vi "S8300E_BootupTime_Delay.vi"() -> ()   [LabVIEW 2011]
uses:
  Instance           3 28Saved   KT55_WaitBootUP_Time .vi
panel:
  out "Begin Time":u32
  out "倒數進度%":u8(slide) scale=0.0..100.0
  out "count down Sec":dbl
  out "系統定義到數秒數":string
  out "System Start Time":u32
  # "S8300E Wait for UUT Ready"
  # "2014-12-15"
  # "Wait for the system Ready\n系統需穩定後才能測試"
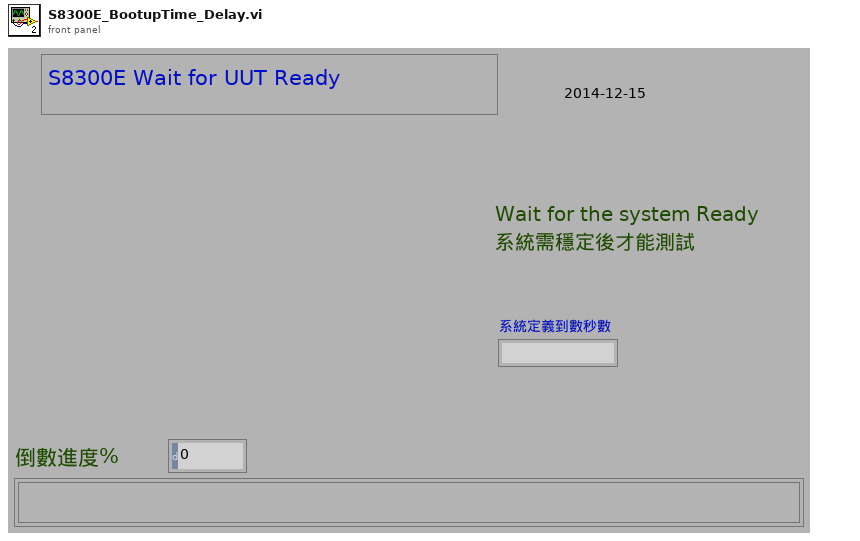
[diagram p1: front panel]
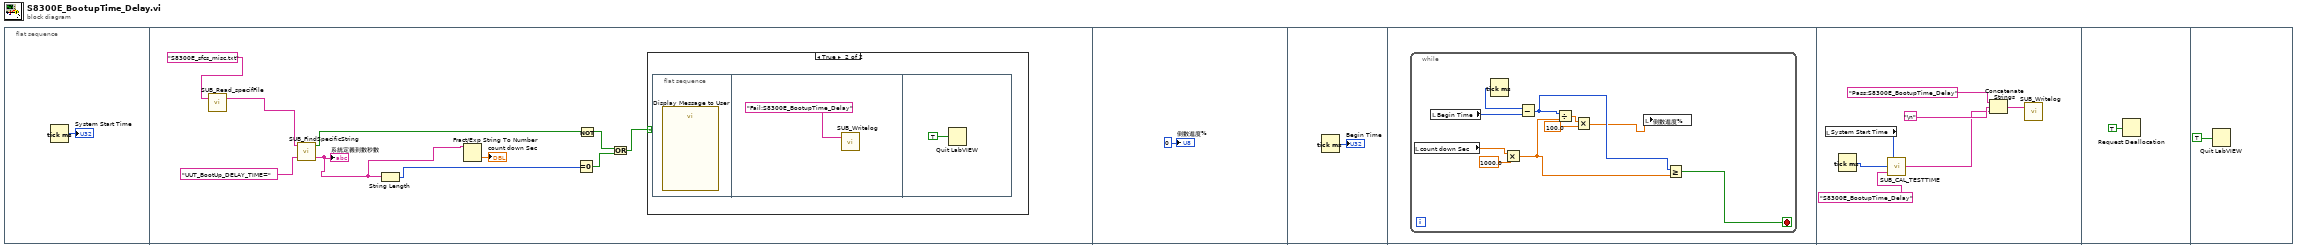
[diagram p0: block diagram]
diagram:
  n1 = flat-sequence {
    frame #0 {
      n2 = Tick Count (ms)() -> (millisecond timer value=→"System Start Time":u32)
    }
    frame #1 {
      n3 = call "SUB_Read_specifFile.vi"("name or relative path"="S8300E_sfcs_misc.txt" ("Script FileName")) -> ("text"=w2:string)  [unwired: 1 in, 1 out]
      n4 = call "SUB_FindSpecificString.vi"("Find this String"="UUT_BootUp_DELAY_TIME=" ("string"), "String data"=w2) -> ("before \"; \" string"=w10:string, "Found"=w7:bool)  [unwired: 2 in]
      "系統定義到數秒數" <- w10
      n5 = String Length(string=w10) -> (length=w8:i32)
      n6 = Fract/Exp String To Number(string=w10) -> (number=→"count down Sec":dbl)  [unwired: 3 in, 1 out]
      n7 = Equal To 0?(x=w8) -> (x = 0?=w5:bool)
      n8 = Not(x=w7) -> (.not. x?=w6:bool)
      n9 = Or(x=w6, y=w5) -> (x .or. y?=w4:bool)
      n10 = case shown="True" w4 {
        frame False {
        }
        frame True {
          n11 = flat-sequence {
            frame #0 {
              n12 = call "Display Message to User"() -> ()  [unwired: 10 in, 2 out]
            }
            frame #1 {
              n13 = call "SUB_Writelog.vi"("Pass/Fail"="Fail:S8300E_BootupTime_Delay") -> ()  [unwired: 2 in]
            }
            frame #2 {
              n14 = Quit LabVIEW(quit? (T)=TRUE) -> ()
            }
          }
        }
      }
    }
    frame #2 {
      "倒數進度%" <- u8 0 ("倒數進度%")
    }
    frame #3 {
      n15 = Tick Count (ms)() -> (millisecond timer value=→"Begin Time":u32)
    }
    frame #4 {
      n16 = while {
        stop <- w16 stop-if-true
        n17 = local read "count down Sec"() -> (w19:dbl)
        n18 = local read "Begin Time"() -> (w18:u32)
        n19 = Tick Count (ms)() -> (millisecond timer value=w24:u32)
        n20 = Multiply(x=w19, y=1000.0) -> (x*y=w20:dbl)
        n21 = Subtract(x=w24, y=w18) -> (x-y=w21:u32)
        n22 = Divide(x=w21, y=w20) -> (x/y=w23:dbl)
        n23 = Multiply(x=w23, y=100.0) -> (x*y=w17:dbl)
        n24 = local write "倒數進度%"(w17) -> ()
        n25 = Greater Or Equal?(x=w21, y=w20) -> (x >= y?=w16:bool)
      }
    }
    frame #5 {
      n26 = local read "System Start Time"() -> (w27:u32)
      n27 = Tick Count (ms)() -> (millisecond timer value=w32:u32)
      n28 = call "SUB_CAL_TESTTIME.vi"("Test Item name"="S8300E_BootupTime_Delay", "Stop tick time"=w32, "Start tick time"=w27) -> ("Test Time output"=w28:string)  [unwired: 2 in]
      n29 = Concatenate Strings("Pass:S8300E_BootupTime_Delay", "\n", w28) -> (w26:string)
      n30 = call "SUB_Writelog.vi"("Pass/Fail"=w26) -> ()  [unwired: 2 in]
    }
    frame #6 {
      n31 = Request Deallocation(TRUE ("flag")) -> ()
    }
    frame #7 {
      n32 = Quit LabVIEW(quit? (T)=TRUE) -> ()
    }
  }
